vi "DAQSampleTime.vi"(0 "Cluster":T4 {"Card Settings"."Start Time" format="%#_3p"; "Card Settings"."End Time" format="%#_3p"; "Card Settings"."Rate" format="%#_3p"}, 5 "First Trigger Time":dbl) -> (14 "Rate":dbl, 15 "Total Samples":i32, 16 "Pre-trigger Samples":i32, 17 "Start Time":dbl, 18 "End Time":dbl, 19 "Samples to remove":i32)   [LabVIEW 2013]
doc: "Translates digitizer times to sampling parameters needed to initialize the daqmx analog input tasks.\nThe start and end times are updated to reflect the actual times which are limited by discrete sampling."
uses:
  Controls/DAQ Card Channel Array.ctl
  Controls/DAQ Channel Settings.ctl
  Controls/DAQ Card Settings.ctl
panel:
  # "Sampling Rate [1/s]"
  # "Start Time [s]"
  # "End Time [s]"
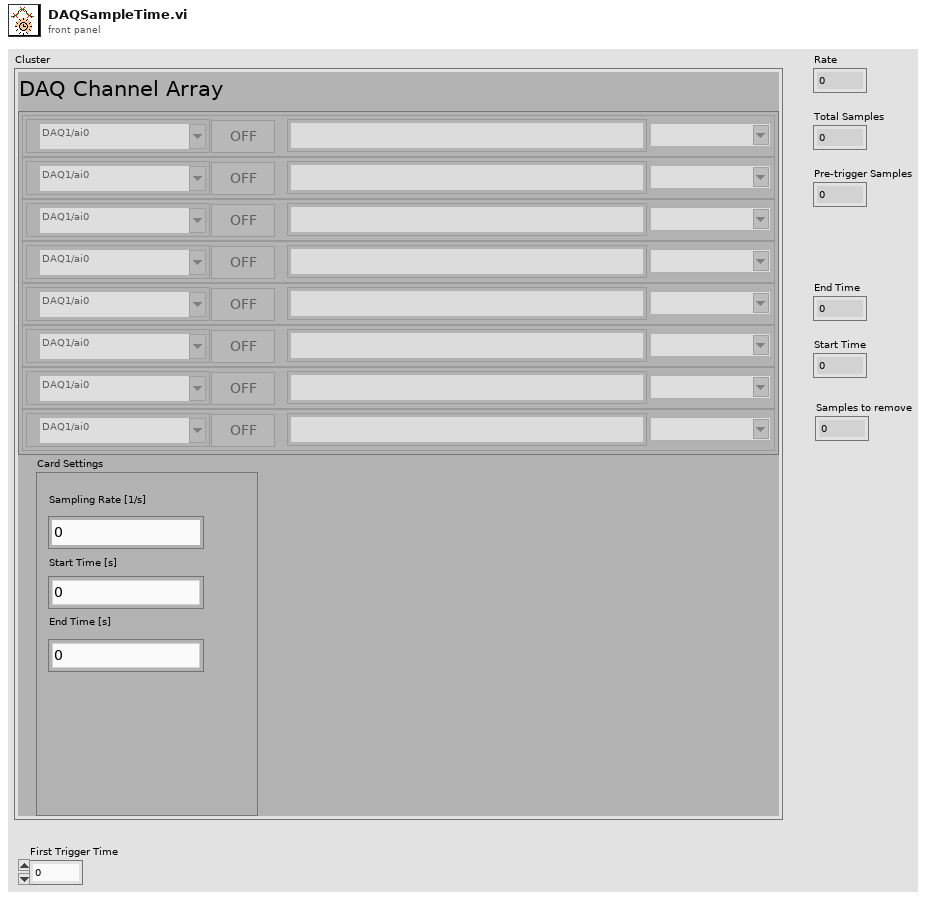
[diagram p1: front panel]
types:
  T1 = typedef "DAQ Card Channel Array.ctl" = T2[]
  T2 = typedef "DAQ Channel Settings.ctl" = cluster{"Active":bool, "Channel Name":string, "Channel":tag, "Voltage Range":string}
  T3 = typedef "DAQ Card Settings.ctl" = cluster{"Rate":dbl, "End Time":dbl, "Start Time":dbl}
  T4 = cluster{"DAQ Channel Array":T1, "Card Settings":T3}
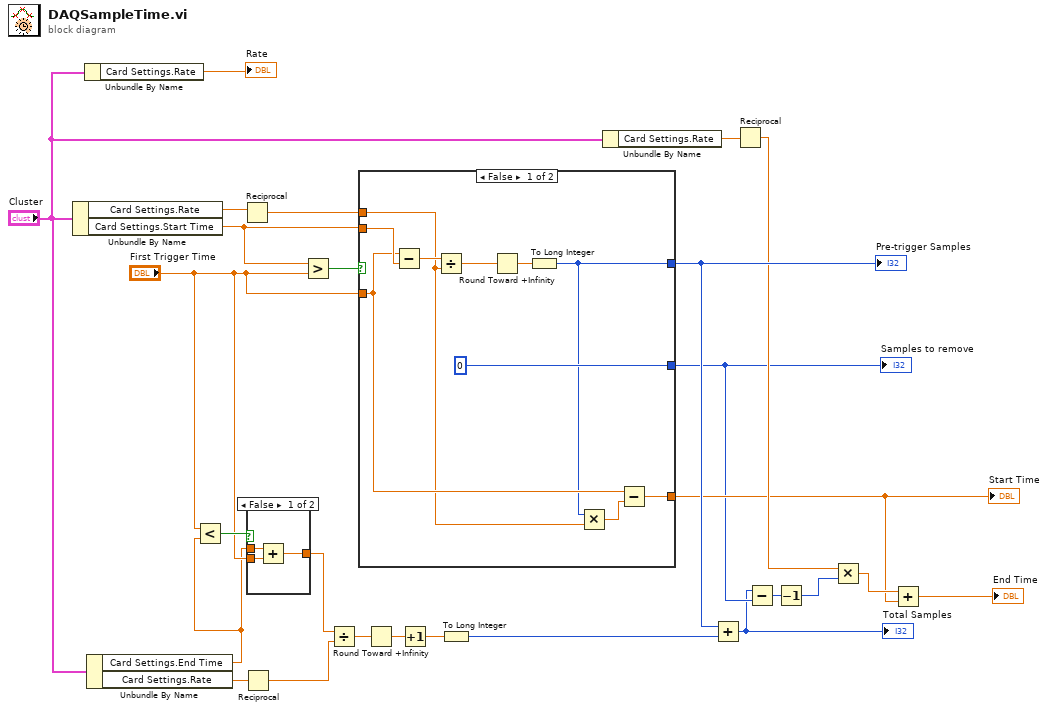
[diagram p0: block diagram]
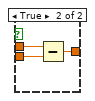
[diagram p2: hidden frame]
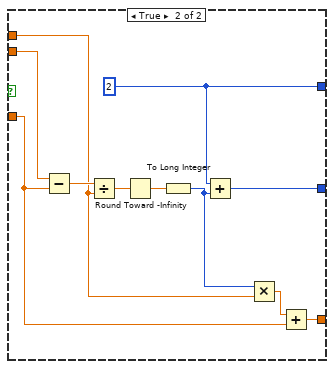
[diagram p3: hidden frame]
diagram:
  n1 = Unbundle By Name("Cluster") -> ("Card Settings.Rate"=w19:dbl, "Card Settings.Start Time"=w25:dbl)
  n2 = Unbundle By Name("Cluster") -> ("Card Settings.Rate"=→"Rate":dbl)
  n3 = Unbundle By Name("Cluster") -> ("Card Settings.End Time"=w1:dbl, "Card Settings.Rate"=w24:dbl)
  n4 = Less?(x="First Trigger Time", y=w1) -> (x < y?=w3:bool)
  n5 = Reciprocal(x=w19) -> (1/x=w20:dbl)
  n6 = Reciprocal(x=w24) -> (1/x=w23:dbl)
  n7 = case shown="False" w3 {
    tunnel: w1 -> [w28 w32]
    tunnel: [w27 w31] -> w22
    tunnel: "First Trigger Time" -> [w29 w30]
    frame False {
      n8 = Add(x=w28, y=w29) -> (x+y=w27:dbl)
    }
    frame True {
      n9 = Subtract(x=w32, y=w30) -> (x-y=w31:dbl)
    }
  }
  n10 = Greater?(x=w25, y="First Trigger Time") -> (0:w26:bool)
  n11 = Divide(x=w22, y=w23) -> (x/y=w21:dbl)
  n12 = case shown="False" w26 {
    tunnel: w25 -> [w38 w53]
    tunnel: "First Trigger Time" -> [w37 w48]
    tunnel: w20 -> [w34 w45]
    tunnel: [w35 w49] -> w16
    tunnel: [0 w46] -> w7
    tunnel: [w33 w43] -> w8
    frame False {
      n13 = Subtract(x=w37, y=w38) -> (x-y=w42:dbl)
      n14 = Divide(x=w42, y=w34) -> (x/y=w41:dbl)
      n15 = Round Toward +Infinity(x=w41) -> (ceil(x): smallest int >= x=w40:dbl)
      n16 = To Long Integer(number=w40) -> (32bit integer=w35:i32)
      n17 = Multiply(x=w35, y=w34) -> (x*y=w36:dbl)
      n18 = Subtract(x=w37, y=w36) -> (x-y=w33:dbl)
    }
    frame True {
      w49 = 2 ("Pre-trigger Samples")
      n19 = Subtract(x=w53, y=w48) -> (x-y=w52:dbl)
      n20 = Divide(x=w52, y=w45) -> (x/y=w51:dbl)
      n21 = Round Toward -Infinity(1:w51) -> (0:w50:dbl)
      n22 = To Long Integer(number=w50) -> (32bit integer=w44:i32)
      n23 = Add(x=w49, y=w44) -> (x+y=w46:i32)
      n24 = Multiply(x=w44, y=w45) -> (x*y=w47:dbl)
      n25 = Add(x=w47, y=w48) -> (x+y=w43:dbl)
    }
  }
  "Start Time" <- w8
  "Pre-trigger Samples" <- w16
  "Samples to remove" <- w7
  n26 = Round Toward +Infinity(x=w21) -> (ceil(x): smallest int >= x=w11:dbl)
  n27 = Increment(x=w11) -> (x+1=w10:dbl)
  n28 = To Long Integer(number=w10) -> (32bit integer=w9:i32)
  n29 = Unbundle By Name("Cluster") -> ("Card Settings.Rate"=w17:dbl)
  n30 = Add(x=w16, y=w9) -> (x+y=w6:i32)
  "Total Samples" <- w6
  n31 = Reciprocal(x=w17) -> (1/x=w15:dbl)
  n32 = Subtract(x=w6, y=w7) -> (x-y=w5:i32)
  n33 = Decrement(x=w5) -> (x-1=w4:i32)
  n34 = Multiply(x=w15, y=w4) -> (x*y=w13:dbl)
  n35 = Add(x=w13, y=w8) -> (x+y=→"End Time":dbl)
